vi "Setup.vi"(7 "Actor in":refnum<class "Actor.lvclass">, 9 "Actor Ref":refnum<vi>, 10 "Spawn":T1) -> (0 "Error out":errorcluster, 2 "Event Ref":refnum<event-registration>, 5 "Actor out":refnum<class "Actor.lvclass">)   [LabVIEW 2025, in "jettl.lvlib" / "Actor.lvlib"]
uses:
  Actor.lvlib
  Actor/Actor.lvclass
  Msg/Msg.lvclass
  Spawn.ctl
  Attributes/Attributes/Attributes.lvclass
  Setup.ctl
  Msg Set.ctl
  Lifecycle.ctl
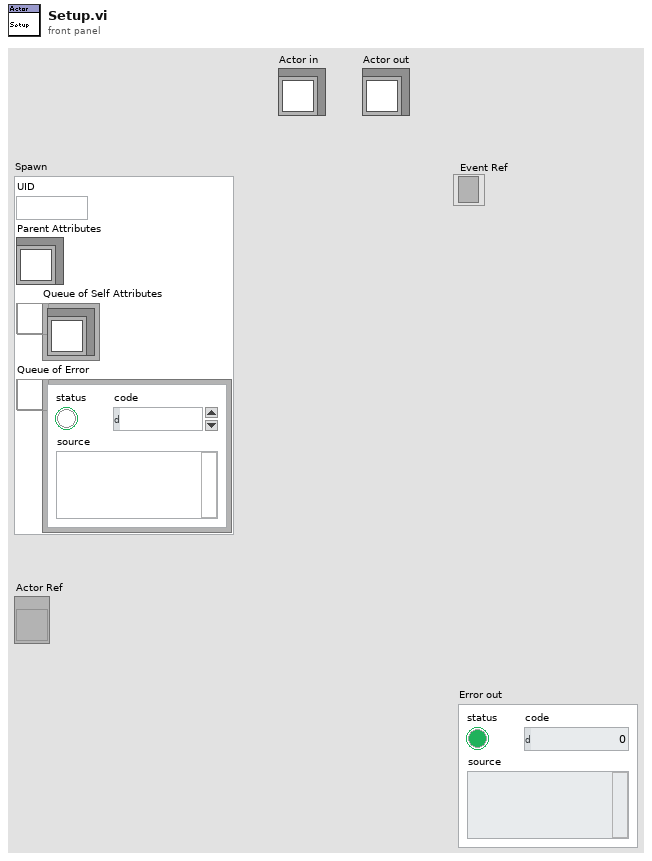
[diagram p1: front panel]
types:
  T1 = typedef "jettl.lvlib/Actor.lvlib/Spawn.ctl" = cluster{"UID":string, "Parent Attributes":refnum<class "Attributes.lvclass">, "Queue of Self Attributes":refnum<queue>, "Queue of Error":refnum<queue>}
  T2 = typedef "jettl.lvlib/Actor.lvlib/Setup.ctl" = cluster{"Unified Msg Set":T3, "UID":string, "Parent Attributes":refnum<class "Attributes.lvclass">, "Queue of Self Attributes":refnum<queue>, "Actor Ref":refnum<vi>}
  T3 = typedef "jettl.lvlib/Actor.lvlib/Msg Set.ctl" = set{refnum<class "Msg.lvclass">}
  T4 = typedef "jettl.lvlib/Actor.lvlib/Lifecycle.ctl" = enum16{"Setup", "Teardown"}
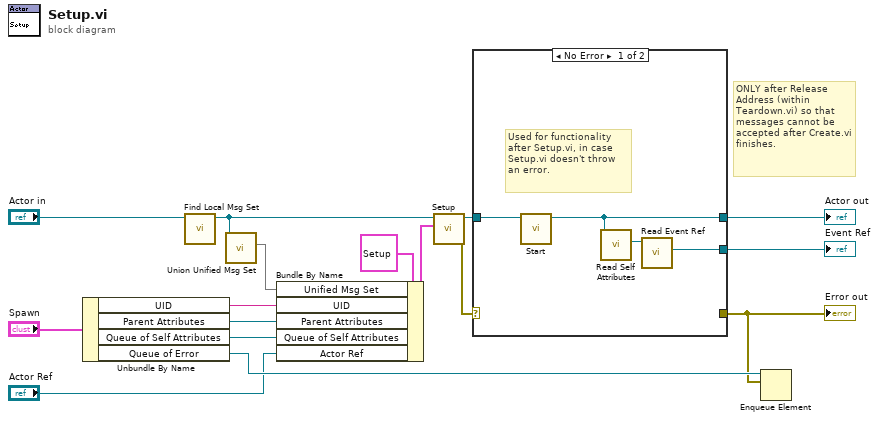
[diagram p0: block diagram]
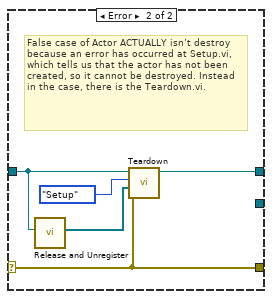
[diagram p2: hidden frame]
diagram:
  # "ONLY after Release Address (within Teardown.vi) so that messages cannot be accepted after Create.vi finishes."
  n1 = Unbundle By Name("Spawn") -> ("UID"=w1:string, "Parent Attributes"=w2:refnum<class "Attributes.lvclass">, "Queue of Self Attributes"=w3:refnum<queue>, "Queue of Error"=w9:refnum<queue>)
  n2 = call-dynamic "Find Local Msg Set.vi"("Actor in"="Actor in") -> ("Actor out"=w15:refnum<class "Actor.lvclass">)  [unwired: 10 in]
  n3 = call-dynamic "Union Unified Msg Set.vi"("Get Actor in"=w15) -> ("Unified Msg Set"=w5:T3)  [unwired: 10 in]
  n4 = Bundle By Name(cluster=T2 {"Unified Msg Set"={}, "UID"="", "Parent Attributes"=refnum, "Queue of Self Attributes"=refnum, "Actor Ref"=refnum} ("Setup"), "Unified Msg Set"=w5, "UID"=w1, "Parent Attributes"=w2, "Queue of Self Attributes"=w3, "Actor Ref"="Actor Ref") -> (w6:T2)
  n5 = call-dynamic "Setup.vi"("Setup"=w6, "Actor in"=w15) -> ("Error out"=w12:errorcluster, "Actor out"=w14:refnum<class "Actor.lvclass">)  [unwired: 8 in]
  n6 = case shown="No Error" w12 {
    selector: w12 -> [_ w22]
    tunnel: w14 -> [w18 w24]
    tunnel: [w19 _] -> w11
    tunnel: [_ w22] -> w8
    tunnel: [w17 w23] -> w13
    frame No Error {
      # "Used for functionality after Setup.vi, in case Setup.vi doesn't throw an error."
      n7 = call-dynamic "Start.vi"("Actor in"=w18) -> ("Actor out"=w17:refnum<class "Actor.lvclass">)  [unwired: 10 in]
      n8 = call-dynamic "Read Self Attributes.vi"("Actor in"=w17) -> ("Self Attributes"=w20:refnum<class "Attributes.lvclass">)  [unwired: 10 in]
      n9 = call-dynamic "Read Event Ref.vi"("Attributes in"=w20) -> ("Event Ref"=w19:refnum<event-registration>)  [unwired: 10 in]
    }
    frame Error {
      # "False case of Actor ACTUALLY isn’t destroy because an error has occurred at Setup.vi, which tells us that the actor has not been created, so it cannot be destroyed. Instead in the case, there is the Teardown.vi."
      n10 = call "Release and Unregister.vi"("Actor"=w24) -> ("Unhandled Msgs"=w25:refnum<class "Msg.lvclass">[])  [unwired: 10 in]
      n11 = call-dynamic "Teardown.vi"("Error in"=w22, "Unhandled Msgs"=w25, "Lifecycle"=Lifecycle."Setup", "Actor in"=w24) -> ("Actor out"=w23:refnum<class "Actor.lvclass">)  [unwired: 7 in]
    }
  }
  "Actor out" <- w13
  "Error out" <- w8
  "Event Ref" <- w11
  n12 = Enqueue Element(queue=w9, element=w8) -> ()  [unwired: 2 in, 3 out]
